vi "T10.vi"(2 "Parametry Ziemi":T1={"a - półoś duża"=6378137.0, "b - półoś mała"=6356752.3141999999998} {"b - półoś mała" format="%_20f"; "a - półoś duża" format="%_20g"}, 3 "fi'":ext) -> (7 "T10":ext)   [LabVIEW 2015, in "Biblioteka moduł map v3.lvlib" / "Konwersja wsp.lvlib" / "UTM.lvlib" / "Konwersja z UTM na wsp geograficzne.lvlib"]
uses:
  Konwersja z UTM na wsp geograficzne.lvlib
  UTM.lvlib
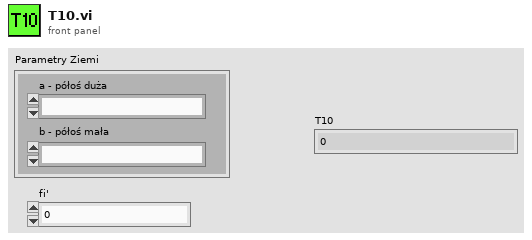
[diagram p1: front panel]
types:
  T1 = cluster{"a - półoś duża":ext, "b - półoś mała":ext}
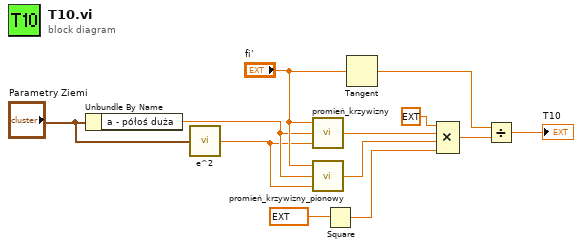
[diagram p0: block diagram]
diagram:
  n1 = Unbundle By Name("Parametry Ziemi") -> ("a - półoś duża"=w3:ext)
  n2 = call "e^2.vi"("Parametry Ziemi"="Parametry Ziemi") -> ("e^2"=w1:ext)  [unwired: 4 in]
  n3 = call "promień_krzywizny.vi"("e^2"=w1, "a"=w3, "fi[rad]"="fi'") -> ("Promien krzywizny południka"=w6:ext)  [unwired: 2 in]
  n4 = call "promień_krzywizny_pionowy.vi"("e^2"=w1, "a"=w3, "fi[rad]"="fi'") -> ("Promien krzywizny równoleżnika"=w5:dbl)  [unwired: 2 in]
  n5 = Square(x=ext 0.9996 ("k0")) -> (x^2=w7:ext)
  n6 = Tangent(1:"fi'") -> (0:w9:ext)
  n7 = Compound Arithmetic op=MULTIPLY(ext 2.0 ("value"), w6, w5, w7) -> (w12:ext)
  n8 = Divide(x=w9, y=w12) -> (x/y=→"T10":ext)
